vi "Example.SubChat.vi"() -> ()   [LabVIEW 2025]
uses:
  libzmq-v143-mt-4_3_6/libzmq-v143-mt-4_3_6.lvlib
  libzmq-v143-mt-4_3_6/ctls/SocketType.ctl
  libzmq-v143-mt-4_3_6/ctls/SocketOption.ctl
panel:
  in  "stop":bool
  out "error out":errorcluster
  out "buf out":string
  in  "TCP":bool=TRUE
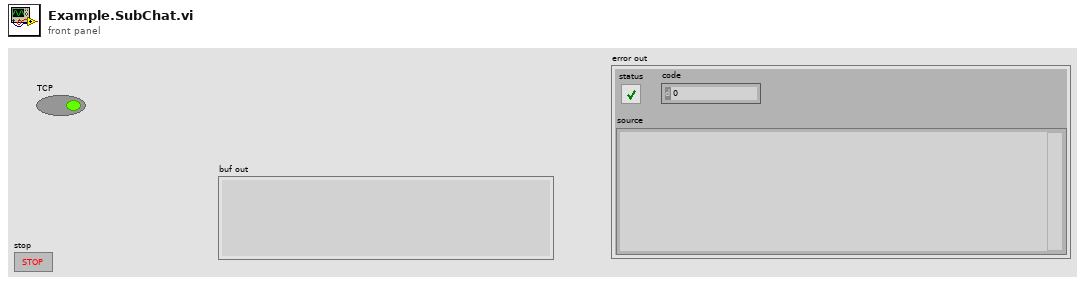
[diagram p1: front panel]
types:
  T1 = typedef "libzmq-v143-mt-4_3_6.lvlib/SocketOption.ctl" = enum8{"NONE", "ZMQ_HWM", "<2>", "ZMQ_SWAP", "ZMQ_AFFINITY", "ZMQ_ROUTING_ID", "ZMQ_SUBSCRIBE", "ZMQ_UNSUBSCRIBE", "ZMQ_RATE", "ZMQ_RECOVERY_IVL", "ZMQ_MCAST_LOOP", "ZMQ_SNDBUF", "ZMQ_RCVBUF", "ZMQ_RCVMORE", "ZMQ_FD", "ZMQ_EVENTS", "ZMQ_TYPE", "ZMQ_LINGER", "ZMQ_RECONNECT_IVL", "ZMQ_BACKLOG", "ZMQ_RECOVERY_IVL_MSEC", "ZMQ_RECONNECT_IVL_MAX", "ZMQ_MAXMSGSIZE", "ZMQ_SNDHWM", "ZMQ_RCVHWM", "ZMQ_MULTICAST_HOPS", "<26>", "ZMQ_RCVTIMEO", "ZMQ_SNDTIMEO", "<29>", "<30>", "ZMQ_IPV4ONLY", "ZMQ_LAST_ENDPOINT", "ZMQ_ROUTER_MANDATORY", "ZMQ_TCP_KEEPALIVE", "ZMQ_TCP_KEEPALIVE_CNT", "ZMQ_TCP_KEEPALIVE_IDLE", "ZMQ_TCP_KEEPALIVE_INTVL", "ZMQ_TCP_ACCEPT_FILTER", "ZMQ_IMMEDIATE", "ZMQ_XPUB_VERBOSE", "ZMQ_ROUTER_RAW", "ZMQ_IPV6", "ZMQ_MECHANISM", "ZMQ_PLAIN_SERVER", "ZMQ_PLAIN_USERNAME", "ZMQ_PLAIN_PASSWORD", "ZMQ_CURVE_SERVER", "ZMQ_CURVE_PUBLICKEY", "ZMQ_CURVE_SECRETKEY", "ZMQ_CURVE_SERVERKEY", "ZMQ_PROBE_ROUTER", "ZMQ_REQ_CORRELATE", "ZMQ_REQ_RELAXED", "ZMQ_CONFLATE", "ZMQ_ZAP_DOMAIN", "ZMQ_ROUTER_HANDOVER", "ZMQ_TOS", "ZMQ_IPC_FILTER_PID", "ZMQ_IPC_FILTER_UID", "ZMQ_IPC_FILTER_GID", "ZMQ_CONNECT_ROUTING_ID", "ZMQ_GSSAPI_SERVER", "ZMQ_GSSAPI_PRINCIPAL", "ZMQ_GSSAPI_SERVICE_PRINCIPAL", "ZMQ_GSSAPI_PLAINTEXT", "ZMQ_HANDSHAKE_IVL", "<67>", "ZMQ_SOCKS_PROXY", "ZMQ_XPUB_NODROP", "ZMQ_BLOCKY", "ZMQ_XPUB_MANUAL", "ZMQ_XPUB_WELCOME_MSG", "ZMQ_STREAM_NOTIFY", "ZMQ_INVERT_MATCHING", "ZMQ_HEARTBEAT_IVL", "ZMQ_HEARTBEAT_TTL", "ZMQ_HEARTBEAT_TIMEOUT", "ZMQ_XPUB_VERBOSER", "ZMQ_CONNECT_TIMEOUT", "ZMQ_TCP_MAXRT", "ZMQ_THREAD_SAFE", "<82>", "<83>", "ZMQ_MULTICAST_MAXTPDU", "ZMQ_VMCI_BUFFER_SIZE", "ZMQ_VMCI_BUFFER_MIN_SIZE", "ZMQ_VMCI_BUFFER_MAX_SIZE", "ZMQ_VMCI_CONNECT_TIMEOUT", "ZMQ_USE_FD", "ZMQ_GSSAPI_PRINCIPAL_NAMETYPE", "ZMQ_GSSAPI_SERVICE_PRINCIPAL_NAMETYPE", "ZMQ_BINDTODEVICE", "ZMQ_ZAP_ENFORCE_DOMAIN", "ZMQ_LOOPBACK_FASTPATH", "ZMQ_METADATA", "ZMQ_MULTICAST_LOOP", "ZMQ_ROUTER_NOTIFY"}
  T2 = typedef "libzmq-v143-mt-4_3_6.lvlib/SocketType.ctl" = enum16{"Pair", "Pub", "Sub", "Request", "Reply", "Dealer", "Router", "Pull", "Push", "XPub", "XSub"}
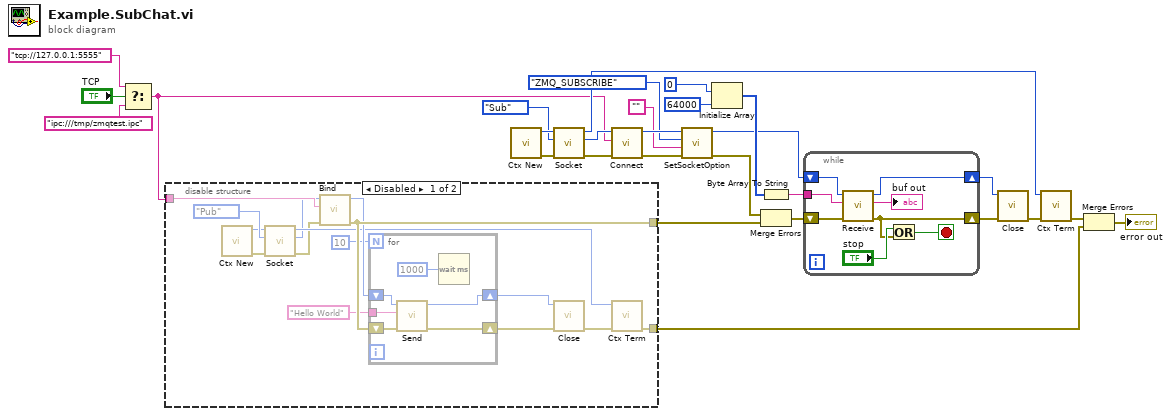
[diagram p0: block diagram]
diagram:
  n1 = Select(t="tcp://127.0.0.1:5555", s="TCP", f="ipc:///tmp/zmqtest.ipc") -> (s? t:f=w11:string)
  n2 = disable-structure shown="Disabled" {
    disable-tunnel: w11 -> [w43 _]
    disable-tunnel: [w42 _] -> w9
    disable-tunnel: [w41 _] -> w7
    frame Disabled {
      n3 = call "Ctx New.vi"() -> ("error out"=w31:errorcluster, "function return"=w32:u64)  [unwired: 10 in]
      n4 = call "Socket.vi"("error in (no error)"=w31, "Socket Type"=SocketType."Pub", "ctx in"=w32) -> ("error out"=w33:errorcluster, "s_"=w34:u64, "ctx out"=w36:u64)  [unwired: 6 in]
      n5 = call "Bind.vi"("error in (no error)"=w33, "addr_"=w43, "s_"=w34) -> ("error out"=w42:errorcluster, "s_ out"=w37:u64)  [unwired: 7 in]
      n6 = for {
        N: 10 -> [_]
        tunnel: "Hello World" -> [w46]
        shift-right: [w48] -> w39
        shift-left: w37 -> [w47]
        shift-right: [w49] -> w40
        shift-left: w42 -> [w45]
        n7 = call "Send.vi"("error in (no error)"=w45, "buf"=w46, "s"=w47) -> ("error out"=w49:errorcluster, "s_"=w48:u64)  [unwired: 7 in]
        n8 = Wait (ms)(milliseconds to wait=u32 1000) -> ()  [unwired: 1 out]
      }
      n9 = call "Close.vi"("error in (no error)"=w40, "s_"=w39) -> ("error out"=w35:errorcluster)  [unwired: 9 in]
      n10 = call "Ctx Term.vi"("error in (no error)"=w35, "context_"=w36) -> ("error out"=w41:errorcluster)  [unwired: 9 in]
    }
    frame Enabled {
    }
  }
  n11 = call "Ctx New.vi"() -> ("error out"=w25:errorcluster, "function return"=w24:u64)  [unwired: 10 in]
  n12 = call "Socket.vi"("error in (no error)"=w25, "Socket Type"=SocketType."Sub", "ctx in"=w24) -> ("error out"=w23:errorcluster, "s_"=w22:u64, "ctx out"=w20:u64)  [unwired: 6 in]
  n13 = call "Connect.vi"("error in (no error)"=w23, "addr_"=w11, "s_"=w22) -> ("error out"=w16:errorcluster, "s_ out"=w4:u64)  [unwired: 7 in]
  n14 = call "SetSocketOption.vi"("error in"=w16, "value"="", "Socket option"=SocketOption."ZMQ_SUBSCRIBE", "socket in"=w4) -> ("error out"=w5:errorcluster, "socket out"=w3:u64)  [unwired: 6 in]
  n15 = Initialize Array(u8 0, 64000 ("dimension size")) -> (w15:u8[])
  n16 = Byte Array To String(unsigned byte array=w15) -> (string=w12:string)
  n17 = Merge Errors(w5, w9) -> (w10:errorcluster)
  n18 = while {
    tunnel: w12 -> [w56]
    shift-right: [w50] -> w17
    shift-left: w10 -> [w54]
    shift-right: [w57] -> w18
    shift-left: w3 -> [w53]
    stop <- w51 stop-if-true
    n19 = call "Receive.vi"("error in (no error)"=w54, "buf in"=w56, "s"=w53) -> ("error out"=w50:errorcluster, "buf out"=→"buf out":string, "s_"=w57:u64)  [unwired: 6 in]
    n20 = Or(x="stop", y=w50) -> (x .or. y?=w51:bool)
  }
  n21 = call "Close.vi"("error in (no error)"=w17, "s_"=w18) -> ("error out"=w21:errorcluster)  [unwired: 9 in]
  n22 = call "Ctx Term.vi"("error in (no error)"=w21, "context_"=w20) -> ("error out"=w8:errorcluster)  [unwired: 9 in]
  n23 = Merge Errors(w8, w7) -> (→"error out":errorcluster)
